vi "Write Cmd ILD1420.vi"(0 "COM port":refnum<visa-resource-name>, 5 "Cmd":T1, 7 "Param1":string, 9 "Param2":string, 11 "Error in":errorcluster) -> (4 "COM port out":refnum<visa-resource-name>, 15 "Error out":errorcluster)   [LabVIEW 2015]
uses:
  Ctls/Cmd_ILD1420.ctl
panel:
  out "return count":u32
  # "PN 11/08/2016"
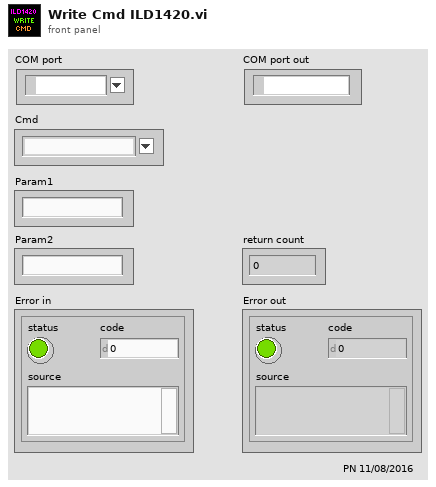
[diagram p1: front panel]
types:
  T1 = typedef "Cmd_ILD1420.ctl" = string
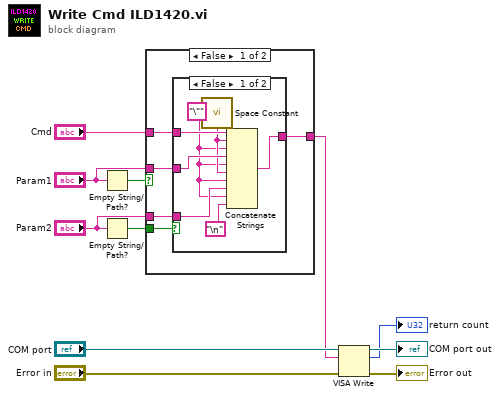
[diagram p0: block diagram]
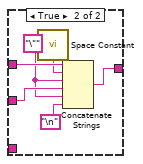
[diagram p2: hidden frame]
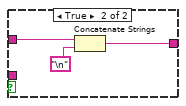
[diagram p3: hidden frame]
diagram:
  n1 = Empty String/Path?(string/path="Param1") -> (empty?=w5:bool)
  n2 = Empty String/Path?(string/path="Param2") -> (empty?=w4:bool)
  n3 = case shown="False" w5 {
    tunnel: "Cmd" -> [w13 w32]
    tunnel: w4 -> [w16 _]
    tunnel: [w12 w30] -> w3
    tunnel: "Param1" -> [w15 _]
    tunnel: "Param2" -> [w14 _]
    frame False {
      n4 = case shown="False" w16 {
        tunnel: w15 -> [w22 w27]
        tunnel: w14 -> [w20 _]
        tunnel: w13 -> [w23 w29]
        tunnel: [w17 w24] -> w12
        frame False {
          w18 = "\""
          n5 = call <vilib>:"Space Constant.vi"() -> ("String"=w21:string)
          n6 = Concatenate Strings(w23, w21, w18, w22, w18, w21, w18, w20, w18, "\n") -> (w17:string)
        }
        frame True {
          w26 = "\""
          n7 = call <vilib>:"Space Constant.vi"() -> ("String"=w28:string)
          n8 = Concatenate Strings(w29, w28, w26, w27, w26, "\n") -> (w24:string)
        }
      }
    }
    frame True {
      n9 = Concatenate Strings(w32, "\n") -> (w30:string)
    }
  }
  n10 = VISA Write(VISA resource name="COM port", write buffer=w3, error in (no error)="Error in") -> (VISA resource name out=→"COM port out":refnum<visa-resource-name>, return count=→"return count":u32, error out=→"Error out":errorcluster)
